vi "Cache.Get Transfers.vi"(11 "Cache in":refnum<class "Cache.lvclass">) -> (2 "Transfers":refnum<class "Transfer.lvclass">[](array[class]), 3 "Cache out":refnum<class "Cache.lvclass">)   [LabVIEW 2017, in "DSF.Engine.lvlib" / "Cache.lvclass"]
uses:
  Cache.lvclass
  Transfer/Transfer.lvclass
  Cache.lvclass/Cache.ctl
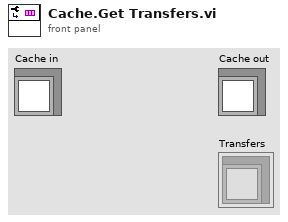
[diagram p1: front panel]
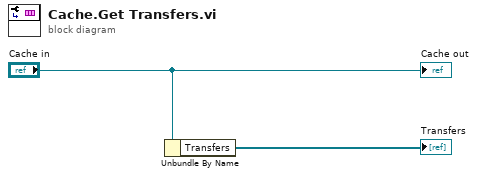
[diagram p0: block diagram]
diagram:
  n1 = Unbundle By Name("Cache in") -> ("Transfers"=→"Transfers":refnum<class "Transfer.lvclass">[])
  "Cache out" <- "Cache in"
